vi "FileUpdater.vi"   [LabVIEW 2014]
uses:
  Robot Global Data.vi
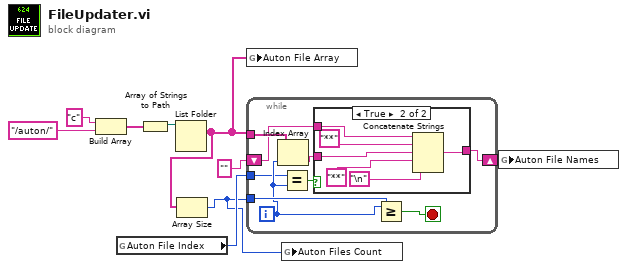
[diagram p0: block diagram]
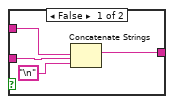
[diagram p2: hidden frame]
diagram:
  n1 = Build Array("c", "/auton/") -> (w5:string[])
  n2 = global read "Robot Global Data.vi" "Auton File Index"() -> (w3:i32)
  n3 = Array of Strings to Path(0:w5) -> (2:w6:path)  [unwired: 1 in]
  n4 = List Folder(path=w6) -> (filenames=w1:string[])  [unwired: 3 in, 3 out]
  n5 = Array Size(array=w1) -> (size(s)=w2:i32)
  n6 = global write "Robot Global Data.vi" "Auton File Array"(w1) -> ()
  n7 = while {
    tunnel: w1 -> [w16]
    tunnel: w2 -> [w17]
    shift-right: [w15] -> w4
    shift-left: "" -> [w14]
    tunnel: w3 -> [w10]
    i -> [w11]
    stop <- w18 stop-if-true
    n8 = Index Array(array=w16, index=w11) -> (element=w13:string)
    n9 = Equal?(x=w10, y=w11) -> (x = y?=w12:bool)
    n10 = case shown="True" w12 {
      tunnel: [w22 w27] -> w15
      tunnel: w14 -> [w19 w24]
      tunnel: w13 -> [w21 w28]
      frame False {
        n11 = Concatenate Strings(w19, w21, "\n") -> (w22:string)
      }
      frame True {
        n12 = Concatenate Strings(w24, "**" ("string"), w28, "**" ("string"), "\n") -> (w27:string)
      }
    }
    n13 = Greater Or Equal?(x=w11, y=w17) -> (x >= y?=w18:bool)
  }
  n14 = global write "Robot Global Data.vi" "Auton Files Count"(w2) -> ()
  n15 = global write "Robot Global Data.vi" "Auton File Names"(w4) -> ()
